vi "Lester Roche programacion 5.vi"() -> ()   [LabVIEW 2011]
panel:
  out "Personas":dbl
  in  "Planta":u16(ring) items=["Planta #1", "Planta #2", "Planta #3"]
  out "A/C":bool
  out "temperatura":i32(slide) scale=0.0..60.0
  # "Se genera la temperatura entre 1-60\nse selecciona la planta usando el menu ring, \nluego se genera el numero de personas entre 1-50"
  # "planta 1 si hay mas de 25 personas y la temperatura\nes mayor a 22 se enciende el A/C\n\nplanta 2 si hay mas de 30 personas y la temperatura\nes mayor a 27 se enciende el A/C\n\nplanta 3 si hay mas de 20 personas y la temperatura\nes mayor a 29 se enciende el A/C"
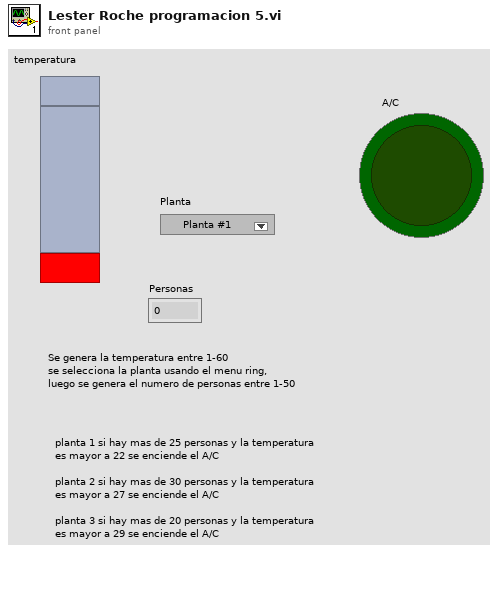
[diagram p1: front panel]
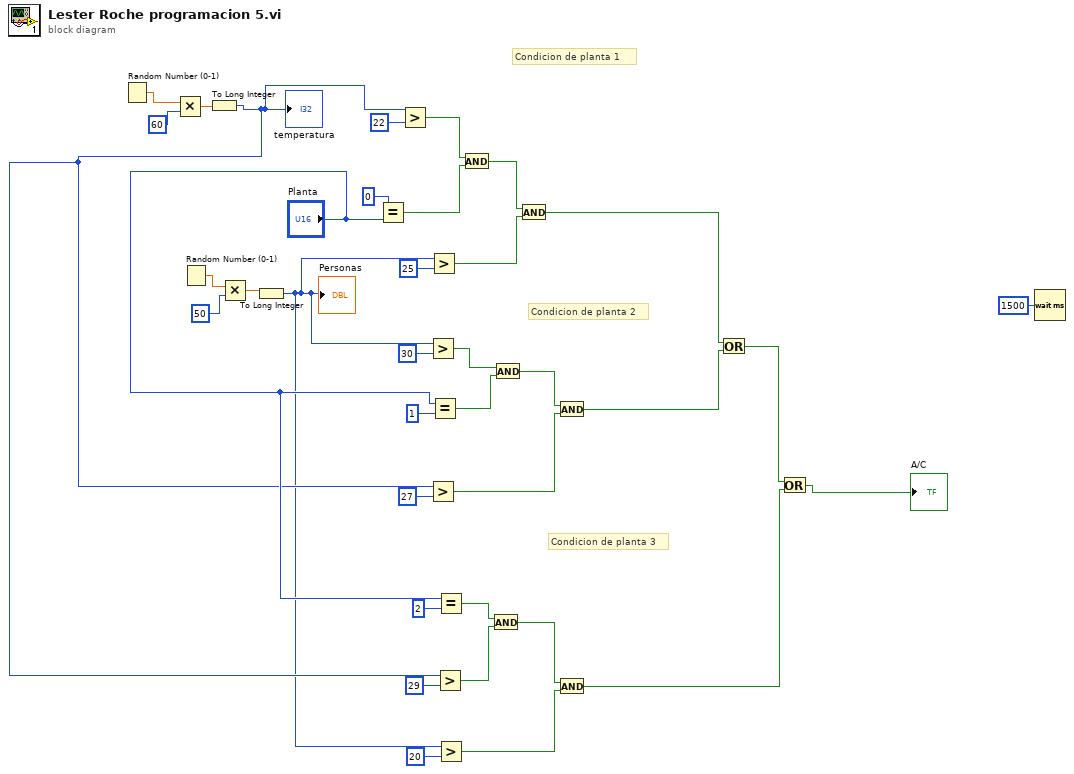
[diagram p0: block diagram]
diagram:
  # "Condicion de planta 3"
  # "Condicion de planta 2"
  # "Condicion de planta 1"
  n1 = Random Number (0-1)() -> (number: 0 to 1=w35:dbl)
  n2 = Multiply(x=w35, y=60) -> (x*y=w33:dbl)
  n3 = Random Number (0-1)() -> (number: 0 to 1=w28:dbl)
  n4 = To Long Integer(number=w33) -> (32bit integer=w9:i32)
  "temperatura" <- w9
  n5 = Multiply(x=w28, y=50) -> (x*y=w26:dbl)
  n6 = To Long Integer(number=w26) -> (32bit integer=w5:i32)
  "Personas" <- w5
  n7 = Equal?(x=0, y="Planta") -> (x = y?=w29:bool)
  n8 = Greater?(x=w9, y=22) -> (0:w30:bool)
  n9 = Greater?(x=w5, y=30) -> (0:w20:bool)
  n10 = Greater?(x=w9, y=27) -> (0:w15:bool)
  n11 = Greater?(x=w5, y=25) -> (0:w23:bool)
  n12 = Equal?(x="Planta", y=u16 1) -> (x = y?=w18:bool)
  n13 = Greater?(x=w9, y=29) -> (0:w7:bool)
  n14 = Equal?(x="Planta", y=u16 2) -> (x = y?=w10:bool)
  n15 = Greater?(x=w5, y=20) -> (0:w3:bool)
  n16 = And(x=w30, y=w29) -> (x .and. y?=w24:bool)
  n17 = And(x=w10, y=w7) -> (x .and. y?=w6:bool)
  n18 = And(x=w20, y=w18) -> (x .and. y?=w17:bool)
  n19 = And(x=w24, y=w23) -> (x .and. y?=w22:bool)
  n20 = And(x=w17, y=w15) -> (x .and. y?=w14:bool)
  n21 = And(x=w6, y=w3) -> (x .and. y?=w2:bool)
  n22 = Or(x=w22, y=w14) -> (x .or. y?=w13:bool)
  n23 = Or(x=w13, y=w2) -> (x .or. y?=→"A/C":bool)
  n24 = Wait (ms)(milliseconds to wait=1500) -> ()  [unwired: 1 out]
